vi "Superimpose Crosshairs.vi"(1 "Merge into Image":bool, 2 "Grid Line Color":u32(colorbox)=16711680, 3 "Refnum in":T1) -> (0 "Refnum out":T1(plugin-control))   [LabVIEW 2023]
uses:
  <vilib>/vision/Image Controls.llb/IMAQ Image.ctl
panel:
  in  "Crosshair size":i32=4
  out "error out":errorcluster
  in  "error in":errorcluster
  # "Set this to true\nto merge the \ncrosshair into\nthe image rather\nthan leaving it \nas a non-destructive\noverlay"
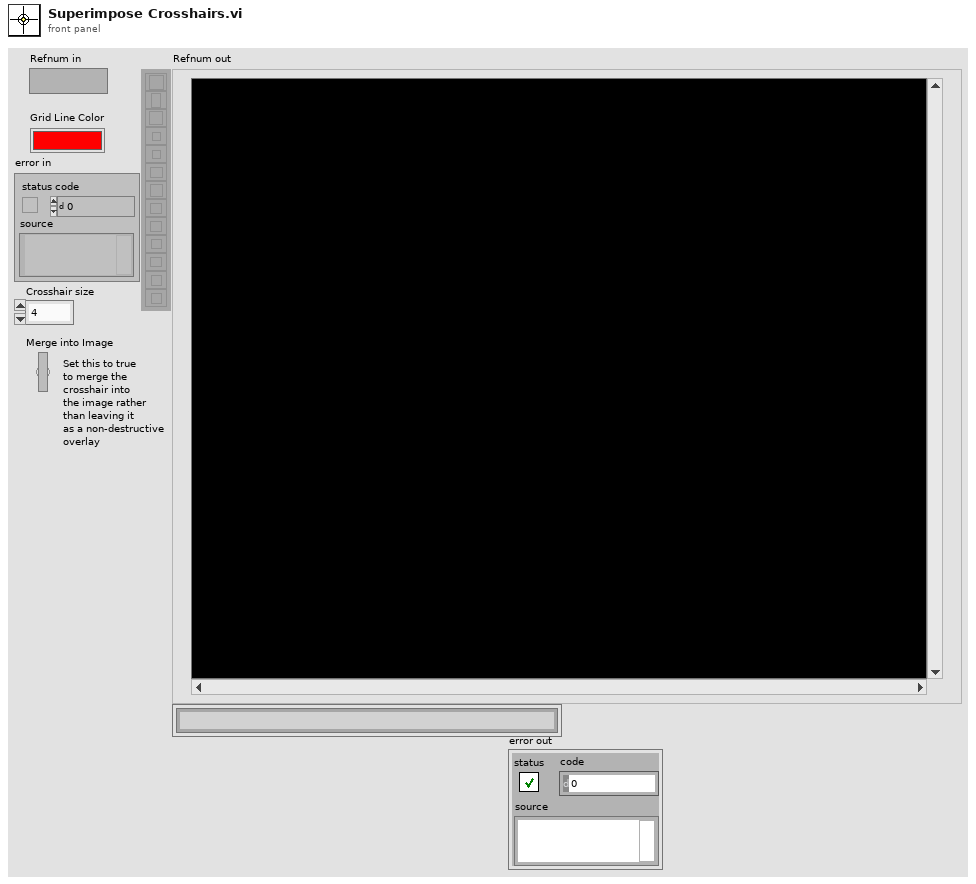
[diagram p1: front panel]
types:
  T1 = typedef "IMAQ Image.ctl" = refnum<image>
  T2 = cluster{"Left":i32, "Top":i32, "Right":i32, "Bottom":i32}
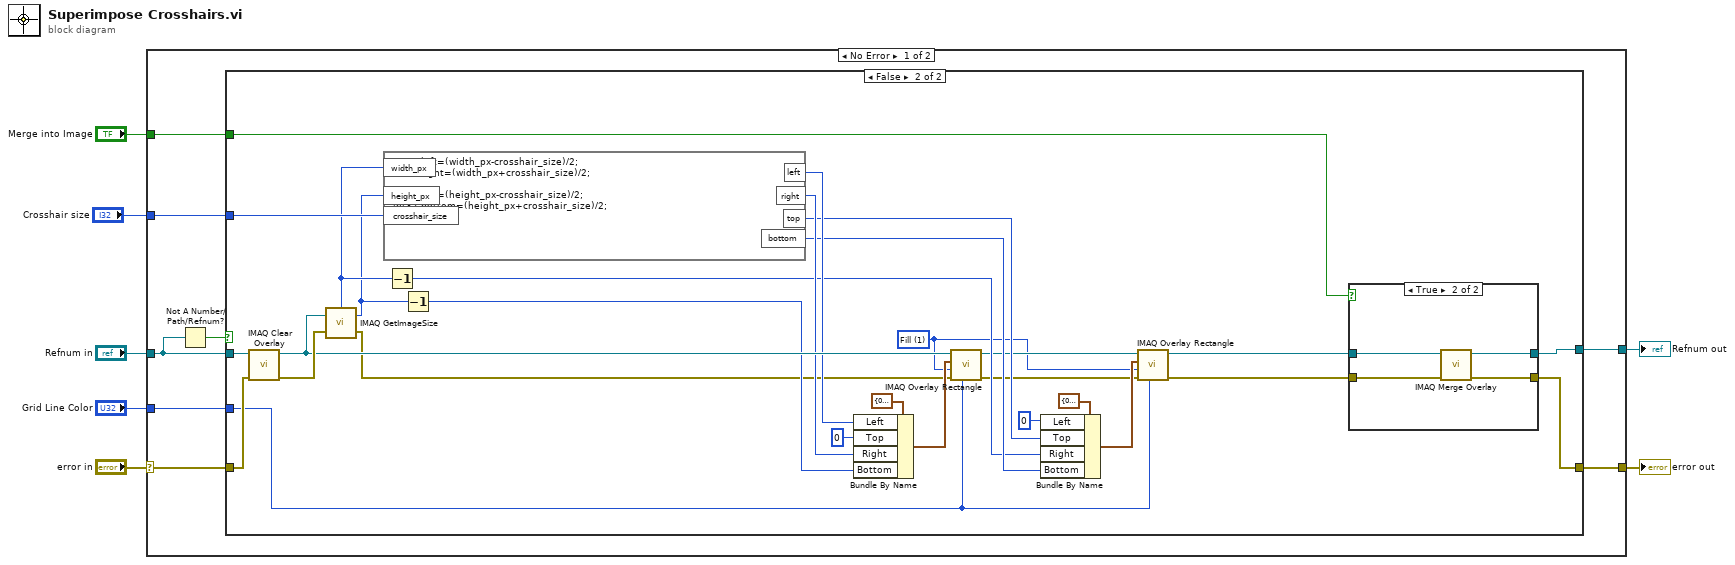
[diagram p0: block diagram]
diagram:
  n1 = case shown="No Error" "error in" {
    selector: "error in" -> [w12 w54]
    tunnel: "Refnum in" -> [w9 w53]
    tunnel: "Grid Line Color" -> [w15 _]
    tunnel: [w14 w53] -> w4
    tunnel: [w13 w54] -> w3
    tunnel: "Merge into Image" -> [w11 _]
    tunnel: "Crosshair size" -> [w10 _]
    frame No Error {
      n2 = Not A Number/Path/Refnum?(number/path/refnum=w9) -> (NaN/Path/Refnum?=w8:bool)
      n3 = case shown="False" w8 {
        tunnel: w15 -> [_ w18]
        tunnel: [w17 w41] -> w14
        tunnel: [w16 w42] -> w13
        tunnel: w9 -> [w17 w46]
        tunnel: w12 -> [w16 w45]
        tunnel: w11 -> [_ w43]
        tunnel: w10 -> [_ w40]
        frame True {
        }
        frame False {
          w19 = u32 1 items=["Frame", "Fill", "Highlight"] ("Drawing Mode (Frame)")
          n4 = call "IMAQ Clear Overlay"("error in (no error)"=w45, "Image"=w46) -> ("error out"=w44:errorcluster, "Image Out"=w39:T1)  [unwired: 8 in]
          n5 = call "IMAQ GetImageSize"("Image"=w39, "error in (no error)"=w44) -> ("Y Resolution"=w32:i32, "X Resolution"=w33:i32, "error out"=w20:errorcluster)  [unwired: 2 in]
          n6 = formula code="int32 left=(width_px-crosshair_size)/2;\nint32 right=(width_px+crosshair_size)/2;\n\nint32 top=(height_px-crosshair_size)/2;\nint32 bottom=(height_px+crosshair_size)/2;"("width_px"=w33, "height_px"=w32, "crosshair_size"=w40) -> ("left"=w37:i32, "right"=w36:i32, "top"=w27:i32, "bottom"=w26:i32)
          n7 = Decrement(x=w33) -> (x-1=w25:i32)
          n8 = Decrement(x=w32) -> (x-1=w31:i32)
          n9 = Bundle By Name(cluster=T2 {"Left"=0, "Top"=0, "Right"=0, "Bottom"=0} ("Rectangle"), "Left"=w37, "Top"=0, "Right"=w36, "Bottom"=w31) -> (w35:T2)
          n10 = call "IMAQ Overlay Rectangle"("Color"=w18, "error in (no error)"=w20, "Drawing Mode (Frame)"=w19, "Rectangle"=w35, "Image"=w39) -> ("error out"=w23:errorcluster, "Image Out"=w24:T1)  [unwired: 5 in]
          n11 = Bundle By Name(cluster=T2 {"Left"=0, "Top"=0, "Right"=0, "Bottom"=0} ("Rectangle"), "Left"=0, "Top"=w27, "Right"=w25, "Bottom"=w26) -> (w29:T2)
          n12 = call "IMAQ Overlay Rectangle"("Color"=w18, "error in (no error)"=w23, "Drawing Mode (Frame)"=w19, "Rectangle"=w29, "Image"=w24) -> ("error out"=w22:errorcluster, "Image Out"=w21:T1)  [unwired: 5 in]
          n13 = case shown="True" w43 {
            tunnel: [w47 w51] -> w42
            tunnel: [w48 w52] -> w41
            tunnel: w22 -> [w47 w50]
            tunnel: w21 -> [w48 w49]
            frame False {
            }
            frame True {
              n14 = call "IMAQ Merge Overlay"("error in (no error)"=w50, "Image Src"=w49) -> ("error out"=w51:errorcluster, "Image Dst Out"=w52:T1)  [unwired: 8 in]
            }
          }
        }
      }
    }
    frame Error {
    }
  }
  "Refnum out" <- w4
  "error out" <- w3
